vi "FTW-Test-JSON-Parallelization.vi"() -> (0 "Test Result":errorcluster)   [LabVIEW 2014]
uses:
  src/core/error/FTW-ERR-ExceptionType.ctl
  src/core/json/FTW-JSON-UpdateMode.ctl
  lib/FTW-LibraryFilepath.vi
  src/core/reflection/FTW-Reflection-Type.vi
  src/core/error/FTW-ERR-ThrowGenericError.vi
  src/core/error/FTW-ERR-ThrowError.vi
  src/core/error/FTW-ERR-CallChain.vi
  src/core/string/FTW-STR-ReplaceWhitespace.vi
  src/core/reflection/FTW-Reflection-Array.vi
  src/core/json/core/FTW-JSON-Core-GetFlattenedValue.vi
  src/core/json/FTW-JSON-Deserialize/FTW-JSON-Deserialize.xnode
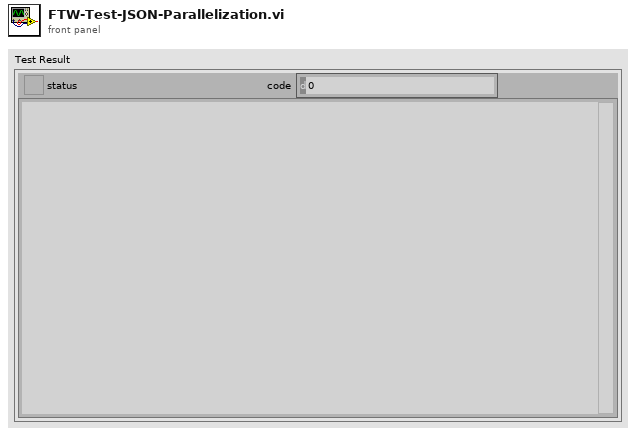
[diagram p1: front panel]
types:
  T1 = cluster{"LoggerDirectory":path, "Value":dbl, "LoggerAddress":string, "BooleanTrue":bool}
  T2 = typedef "FTW-ERR-ExceptionType.ctl" = enum16{"OK", "Info", "Warning", "Error"}
  T3 = typedef "FTW-JSON-UpdateMode.ctl" = enum32{"Upsert", "Update Only", "Insert Only"}
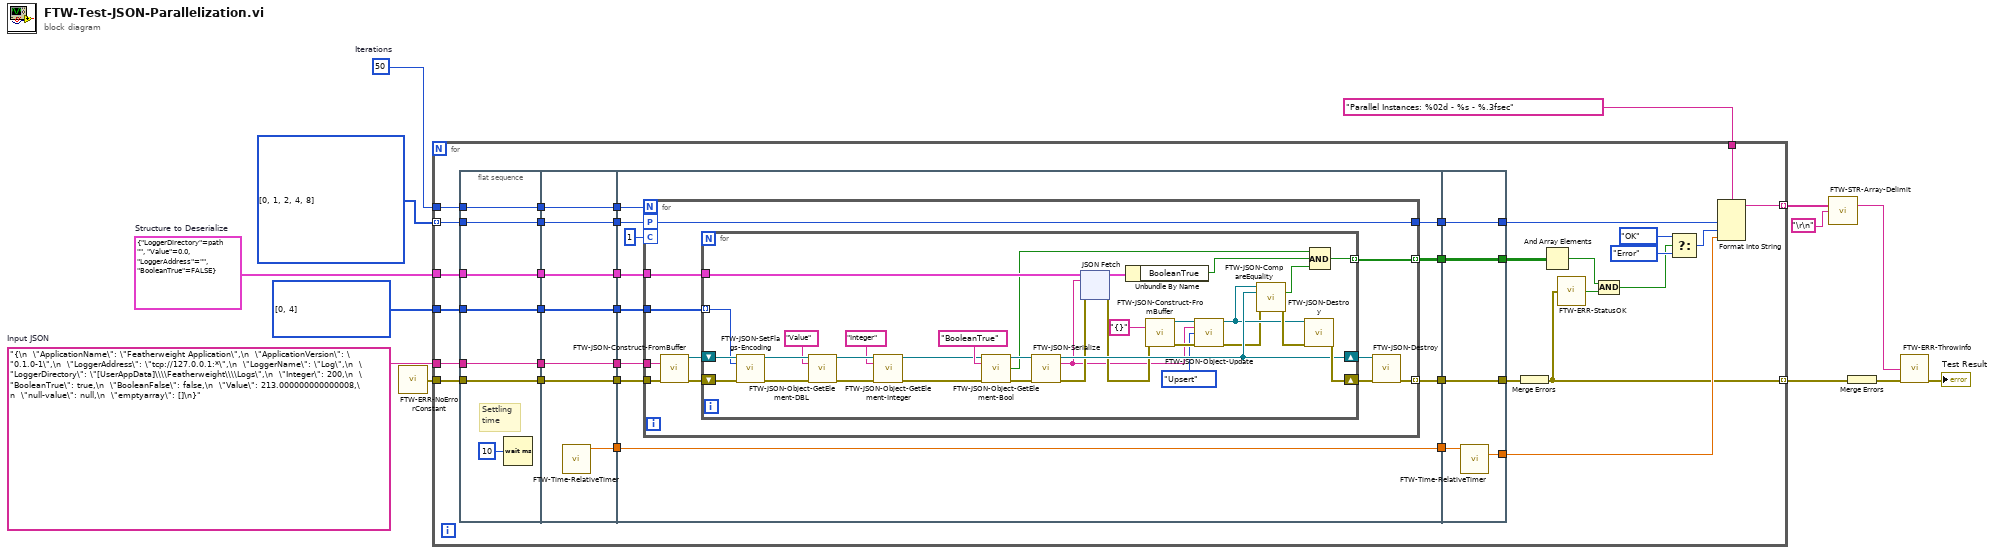
[diagram p0: block diagram]
diagram:
  w9 = T1 {"LoggerDirectory"=path "", "Value"=0.0, "LoggerAddress"="", "BooleanTrue"=FALSE}  # Structure to Deserialize
  w13 = "{\n  \"ApplicationName\": \"Featherweight Application\",\n  \"ApplicationVersion\": \"0.1.0-1\",\n  \"LoggerAddress\": \"tcp://127.0.0.1:*\",\n  \"LoggerName\": \"Log\",\n  \"LoggerDirectory\": \"[UserAppData]\\\\Featherweight\\\\Logs\",\n  \"Integer\": 200,\n  \"BooleanTrue\": true,\n  \"BooleanFalse\": false,\n  \"Value\": 213.000000000000008,\n  \"null-value\": null,\n  \"emptyarray\": []\n}"  # Input JSON
  w6 = 50  # Iterations
  n1 = call "FTW-ERR-NoErrorConstant.vi"() -> ("no error"=w12:errorcluster)
  n2 = for {
    tunnel: w6 -> [w41]
    tunnel: w13 -> [w40]
    tunnel: w12 -> [w39]
    tunnel: i32[] [0, 4] -> [w38]
    tunnel: i32[] [0, 1, 2, 4, 8] -> [w35] mode=indexing
    tunnel: w9 -> [w25]
    tunnel: "Parallel Instances: %02d - %s - %.3fsec" ("format string") -> [w22]
    tunnel: [w18] -> w3 mode=indexing
    tunnel: [w17] -> w7 mode=indexing
    n3 = flat-sequence {
      tunnel: w35 -> [w52]
      tunnel: w38 -> [w53]
      tunnel: w39 -> [w54]
      tunnel: w40 -> [w55]
      tunnel: w41 -> [w56]
      tunnel: [w56] -> w31
      tunnel: [w55] -> w30
      tunnel: [w54] -> w29
      tunnel: [w53] -> w28
      tunnel: [w52] -> w27
      tunnel: w25 -> [w50]
      tunnel: [w50] -> w24
      tunnel: [w63] -> w49
      tunnel: [w62] -> w48
      tunnel: [w61] -> w47
      tunnel: [w60] -> w46
      tunnel: [w59] -> w45
      tunnel: [w58] -> w37
      tunnel: w31 -> [w63]
      tunnel: w30 -> [w62]
      tunnel: w29 -> [w61]
      tunnel: w28 -> [w60]
      tunnel: w27 -> [w58]
      tunnel: w24 -> [w57]
      tunnel: [w57] -> w23
      tunnel: w49 -> [w74]
      tunnel: w48 -> [w66]
      tunnel: w47 -> [w72]
      tunnel: w46 -> [w70]
      tunnel: [w73] -> w44
      tunnel: [w71] -> w43
      tunnel: [w69] -> w42
      tunnel: w45 -> [w69]
      tunnel: w37 -> [w68]
      tunnel: [w67] -> w26
      tunnel: w23 -> [w65]
      tunnel: [w153] -> w34
      tunnel: [w154] -> w36
      tunnel: w44 -> [w154]
      tunnel: w43 -> [w153]
      tunnel: w42 -> [w152]
      tunnel: [w151] -> w19
      tunnel: [w150] -> w21
      tunnel: w26 -> [w150]
      frame #0 {
        # "Settling\ntime"
        n4 = Wait (ms)(milliseconds to wait=u32 10) -> ()  [unwired: 1 out]
      }
      frame #1 {
        n5 = call "FTW-Time-RelativeTimer.vi"() -> ("Current Time"=w59:dbl)  [unwired: 13 in, 2 out]
      }
      frame #2 {
        n6 = for {
          N: w74 -> [_]
          tunnel: w66 -> [w83]
          tunnel: [w77] -> w71 mode=indexing
          tunnel: w70 -> [w78]
          workers-P: w68 -> [w76]
          tunnel: w72 -> [w85]
          tunnel: [w84] -> w73 mode=indexing
          tunnel: [w76] -> w67
          tunnel: w65 -> [w75]
          chunk-C: 1 -> [_]
          n7 = call "FTW-JSON-Construct-FromBuffer.vi"("JSON String (UTF-8)"=w83, "error in"=w85) -> ("JSON Object"=w79:refnum<data-value>, "error out"=w80:errorcluster)  [unwired: 12 in]
          n8 = for {
            tunnel: w78 -> [w113] mode=indexing
            shift-right: [w112] -> w81
            shift-left: w79 -> [w114]
            shift-right: [w117] -> w82
            shift-left: w80 -> [w115]
            tunnel: [w106] -> w77 mode=indexing
            tunnel: w75 -> [w109]
            n9 = call "FTW-JSON-SetFlags-Encoding.vi"("JSON Object"=w114, "Indent Spaces"=w113, "error in"=w115) -> ("JSON Object out"=w108:refnum<data-value>, "error out"=w107:errorcluster)  [unwired: 11 in]
            n10 = call "FTW-JSON-Object-GetElement-DBL.vi"("JSON Object"=w108, "Key"="Value", "error in"=w107) -> ("JSON Object out"=w93:refnum<data-value>, "error out"=w91:errorcluster)  [unwired: 9 in, 2 out]
            n11 = call "FTW-JSON-Object-GetElement-Integer.vi"("JSON Object"=w93, "Key"="Integer", "error in"=w91) -> ("JSON Object out"=w92:refnum<data-value>, "error out"=w90:errorcluster)  [unwired: 9 in, 2 out]
            n12 = call "FTW-JSON-Object-GetElement-Bool.vi"("JSON Object"=w92, "Key"="BooleanTrue", "error in"=w90) -> ("JSON Object out"=w105:refnum<data-value>, "Value"=w94:bool, "error out"=w104:errorcluster)  [unwired: 9 in, 1 out]
            n13 = call "FTW-JSON-Serialize.vi"("JSON Object"=w105, "error in"=w104) -> ("JSON Object out"=w112:refnum<data-value>, "JSON String (UTF-8)"=w96:string, "error out"=w111:errorcluster)  [unwired: 11 in]
            n14 = xnode "JSON Fetch"("Type and Defaults"=w109, "JSON String"=w96, "error in"=w111) -> ("Values"=w87:T1, "error out"=w110:errorcluster)  [unwired: 1 in]
            n15 = Unbundle By Name(w87) -> ("BooleanTrue"=w86:bool)
            n16 = call "FTW-JSON-Construct-FromBuffer.vi"("JSON String (UTF-8)"="{}", "error in"=w110) -> ("JSON Object"=w100:refnum<data-value>, "error out"=w98:errorcluster)  [unwired: 12 in]
            n17 = call "FTW-JSON-Object-Update.vi"("JSON Object"=w100, "JSON Object to Merge"=w96, "Update Mode"=FTW-JSON-UpdateMode."Upsert", "error in"=w98) -> ("JSON Object out"=w99:refnum<data-value>, "error out"=w97:errorcluster)  [unwired: 10 in]
            n18 = call "FTW-JSON-CompareEquality.vi"("JSON Object"=w99, "JSON Object to Compare"=w112, "error in"=w97) -> ("Equal?"=w88:bool, "error out"=w116:errorcluster)  [unwired: 10 in, 1 out]
            n19 = call "FTW-JSON-Destroy.vi"("JSON Object"=w99, "error in"=w116) -> ("error out"=w117:errorcluster)  [unwired: 13 in]
            n20 = Compound Arithmetic op=AND(w94, w86, w88) -> (w106:bool)
          }
          n21 = call "FTW-JSON-Destroy.vi"("JSON Object"=w81, "error in"=w82) -> ("error out"=w84:errorcluster)  [unwired: 13 in]
        }
      }
      frame #3 {
        n22 = call "FTW-Time-RelativeTimer.vi"("Previous Time"=w152) -> ("Elapsed Time"=w151:dbl)  [unwired: 12 in, 2 out]
      }
    }
    n23 = Merge Errors(w36) -> (w17:errorcluster)
    n24 = And Array Elements(Boolean array=w34) -> (logical AND=w32:bool)
    n25 = call "FTW-ERR-StatusOK.vi"("error to check"=w17) -> ("Status OK?"=w33:bool)
    n26 = And(x=w32, y=w33) -> (x .and. y?=w14:bool)
    n27 = Select(t=FTW-ERR-ExceptionType."OK" ("Exception"), s=w14, f=FTW-ERR-ExceptionType."Error" ("Exception")) -> (s? t:f=w20:T2)
    n28 = Format Into String(format string=w22, w21, w20, w19) -> (resulting string=w18:string)  [unwired: 2 in, 1 out]
  }
  n29 = call "FTW-STR-Array-Delimit.vi"("Array of Strings"=w3, "Delimiter"="\r\n") -> ("Delimited String"=w2:string)  [unwired: 13 in]
  n30 = Merge Errors(w7) -> (w5:errorcluster)
  n31 = call "FTW-ERR-ThrowInfo.vi"("Informational Message"=w2, "error in"=w5) -> ("error out"=→"Test Result":errorcluster)  [unwired: 13 in]
